vi "InterruptsGroup.vi"(0 "AnalogTriggers":T2[](array[typedef])=[{"InHysteresis"=FALSE, "OverLimit"=FALSE, "Rising"=FALSE, "Falling"=FALSE}, {"InHysteresis"=FALSE, "OverLimit"=FALSE, "Rising"=FALSE, "Falling"=FALSE}, {"InHysteresis"=FALSE, "OverLimit"=FALSE, "Rising"=FALSE, "Falling"=FALSE}, {"InHysteresis"=FALSE, "OverLimit"=FALSE, "Rising"=FALSE, "Falling"=FALSE}, {"InHysteresis"=FALSE, "OverLimit"=FALSE, "Rising"=FALSE, "Falling"=FALSE}, {"InHysteresis"=FALSE, "OverLimit"=FALSE, "Rising"=FALSE, "Falling"=FALSE}, {"InHysteresis"=FALSE, "OverLimit"=FALSE, "Rising"=FALSE, "Falling"=FALSE}, {"InHysteresis"=FALSE, "OverLimit"=FALSE, "Rising"=FALSE, "Falling"=FALSE}], 1 "DigitalInputs":bool[](array[boolean])=[FALSE, FALSE, FALSE, FALSE, FALSE, FALSE, FALSE, FALSE, FALSE, FALSE, FALSE, FALSE, FALSE, FALSE, FALSE, FALSE, FALSE, FALSE, FALSE, FALSE, FALSE, FALSE, FALSE, FALSE, FALSE, FALSE, FALSE, FALSE, FALSE, FALSE, FALSE, FALSE], 2 "SystemTime":u32, 3 "Configs":T3, 4 "Occurances":T1) -> (5 "Timestamps":T5)   [LabVIEW 2019]
uses:
  Controls/Interrupt_Timestamps.ctl
  Controls/Interrupt_Configs.ctl
  Helpers/Source.ctl
  Helpers/AnalogTriggerOutput.ctl
  Controls/Interrupt_Occurances.ctl
  <vilib>/rvi/Emulation/niFpgaSctlEmulationGetInTimedLoop.vi
  <vilib>/rvi/Emulation/niFpgaProcessEmulError.vi
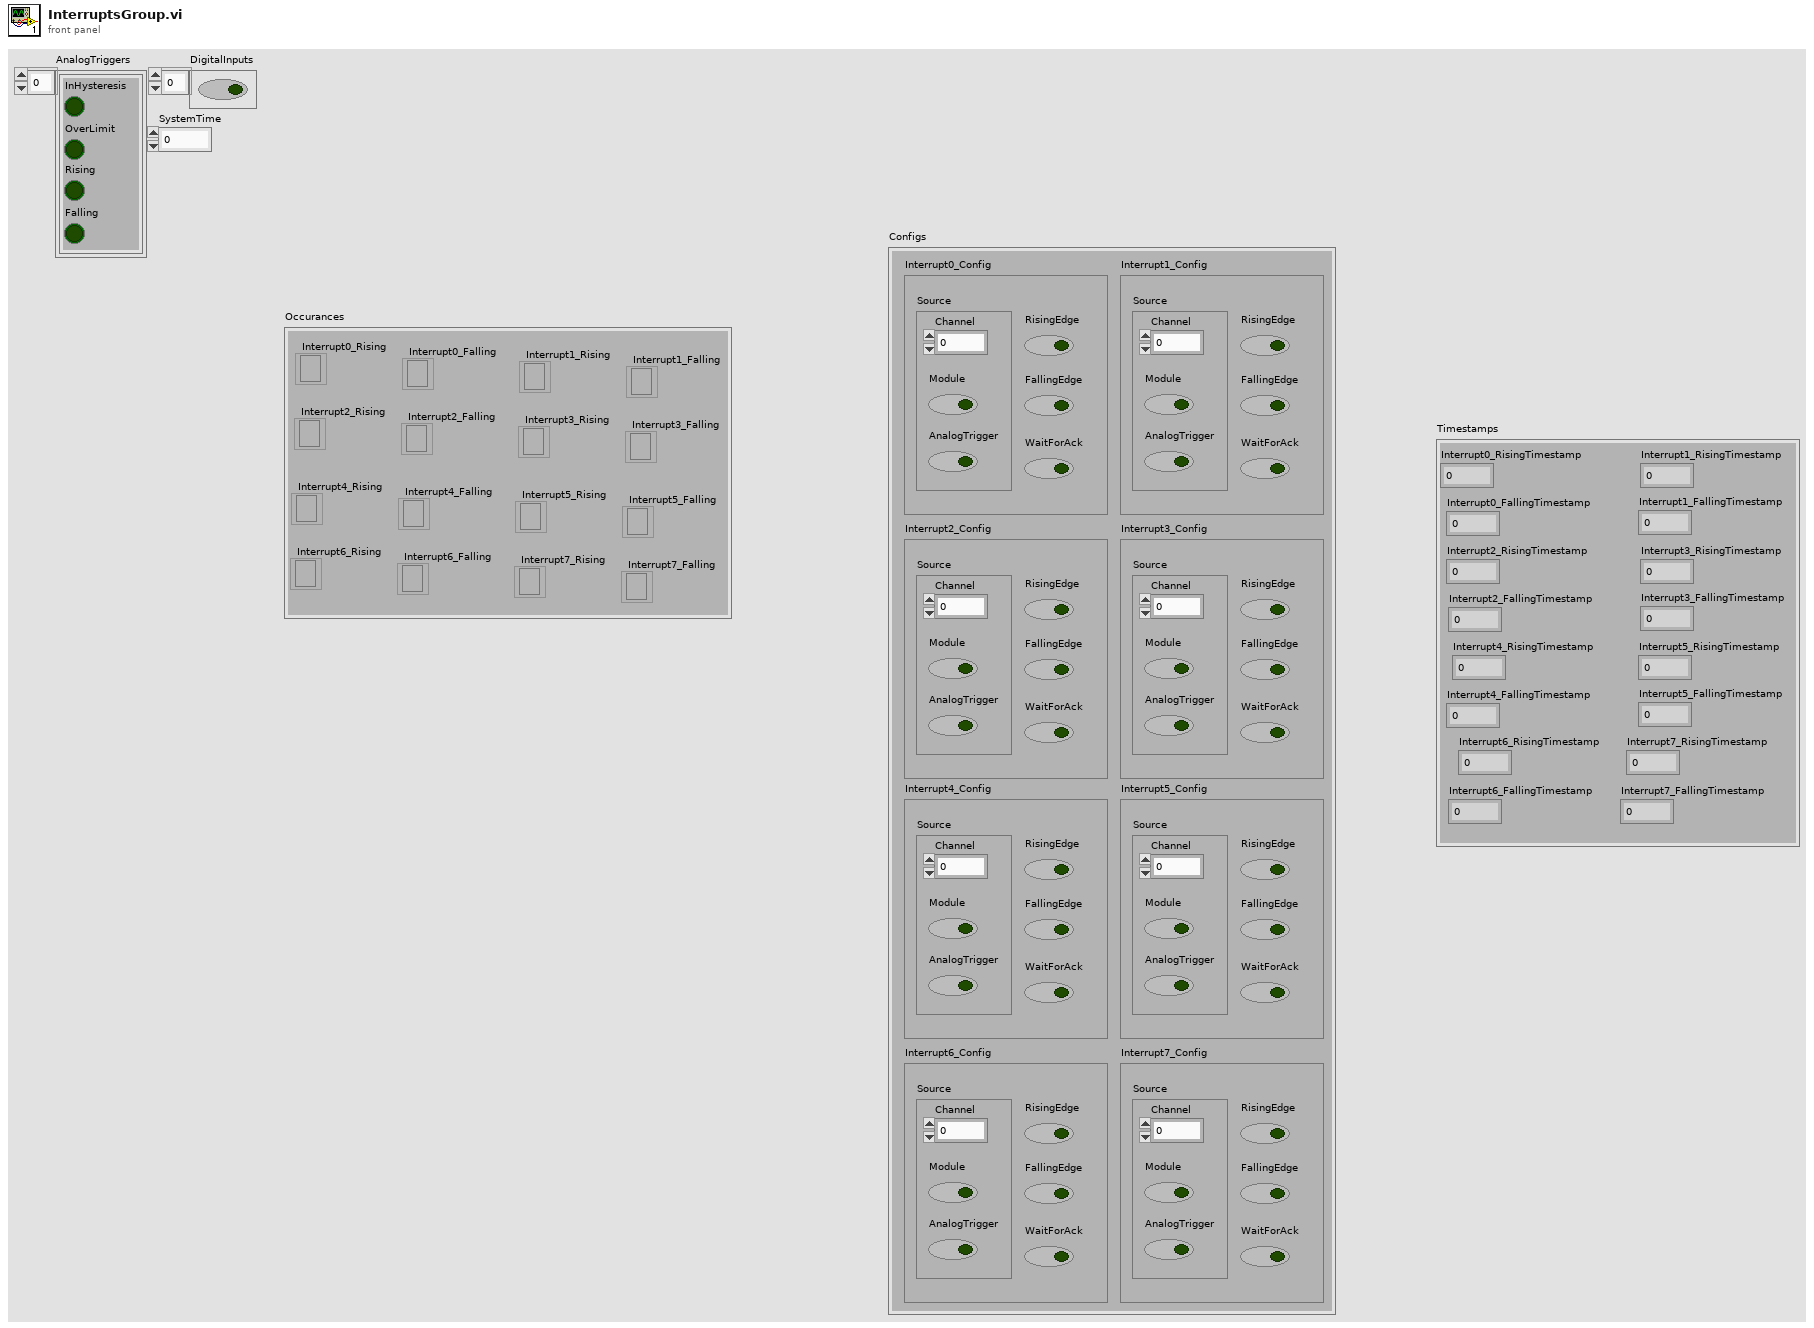
[diagram p1: front panel]
types:
  T1 = typedef "Interrupt_Occurances.ctl" = cluster{"Interrupt0_Rising":refnum<k4>, "Interrupt0_Falling":refnum<k4>, "Interrupt1_Rising":refnum<k4>, "Interrupt1_Falling":refnum<k4>, "Interrupt2_Rising":refnum<k4>, "Interrupt2_Falling":refnum<k4>, "Interrupt3_Rising":refnum<k4>, "Interrupt3_Falling":refnum<k4>, "Interrupt4_Rising":refnum<k4>, "Interrupt4_Falling":refnum<k4>, "Interrupt5_Rising":refnum<k4>, "Interrupt5_Falling":refnum<k4>, "Interrupt6_Rising":refnum<k4>, "Interrupt6_Falling":refnum<k4>, "Interrupt7_Rising":refnum<k4>, "Interrupt7_Falling":refnum<k4>}
  T2 = typedef "AnalogTriggerOutput.ctl" = cluster{"InHysteresis":bool, "OverLimit":bool, "Rising":bool, "Falling":bool}
  T3 = typedef "Interrupt_Configs.ctl" = cluster{"Interrupt0_Config":cluster{"Source":T4, "RisingEdge":bool, "FallingEdge":bool, "WaitForAck":bool}, "Interrupt1_Config":cluster{"Source":T4, "RisingEdge":bool, "FallingEdge":bool, "WaitForAck":bool}, "Interrupt2_Config":cluster{"Source":T4, "RisingEdge":bool, "FallingEdge":bool, "WaitForAck":bool}, "Interrupt3_Config":cluster{"Source":T4, "RisingEdge":bool, "FallingEdge":bool, "WaitForAck":bool}, "Interrupt4_Config":cluster{"Source":T4, "RisingEdge":bool, "FallingEdge":bool, "WaitForAck":bool}, "Interrupt5_Config":cluster{"Source":T4, "RisingEdge":bool, "FallingEdge":bool, "WaitForAck":bool}, "Interrupt6_Config":cluster{"Source":T4, "RisingEdge":bool, "FallingEdge":bool, "WaitForAck":bool}, "Interrupt7_Config":cluster{"Source":T4, "RisingEdge":bool, "FallingEdge":bool, "WaitForAck":bool}}
  T4 = typedef "Source.ctl" = cluster{"Channel":fxp<+,4,4>, "Module":bool, "AnalogTrigger":bool}
  T5 = typedef "Interrupt_Timestamps.ctl" = cluster{"Interrupt0_RisingTimestamp":u32, "Interrupt0_FallingTimestamp":u32, "Interrupt1_RisingTimestamp":u32, "Interrupt1_FallingTimestamp":u32, "Interrupt2_RisingTimestamp":u32, "Interrupt2_FallingTimestamp":u32, "Interrupt3_RisingTimestamp":u32, "Interrupt3_FallingTimestamp":u32, "Interrupt4_RisingTimestamp":u32, "Interrupt4_FallingTimestamp":u32, "Interrupt5_RisingTimestamp":u32, "Interrupt5_FallingTimestamp":u32, "Interrupt6_RisingTimestamp":u32, "Interrupt6_FallingTimestamp":u32, "Interrupt7_RisingTimestamp":u32, "Interrupt7_FallingTimestamp":u32}
  T6 = cluster{"Source":T4, "RisingEdge":bool, "FallingEdge":bool, "WaitForAck":bool}
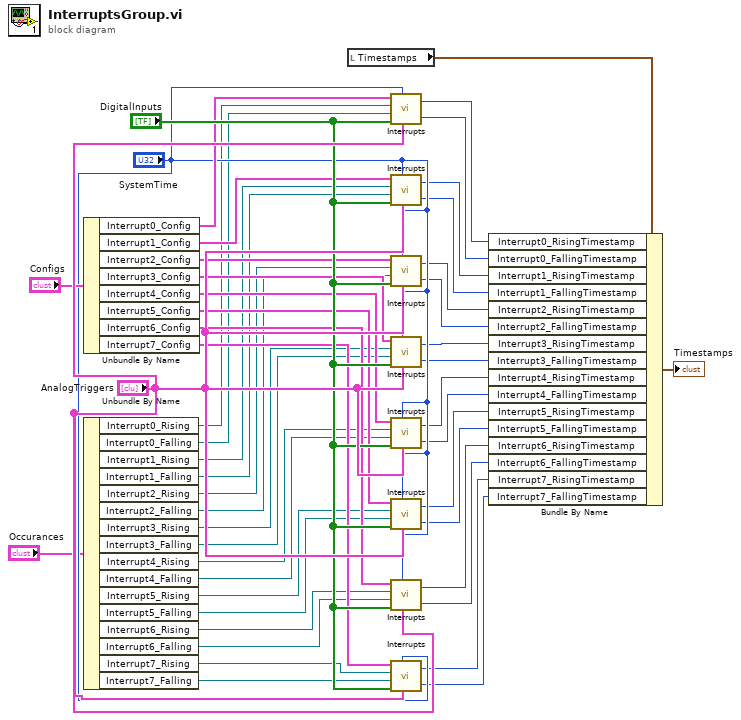
[diagram p0: block diagram]
diagram:
  n1 = Unbundle By Name("Configs") -> ("Interrupt0_Config"=w44:T6, "Interrupt1_Config"=w43:T6, "Interrupt2_Config"=w42:T6, "Interrupt3_Config"=w41:T6, "Interrupt4_Config"=w40:T6, "Interrupt5_Config"=w39:T6, "Interrupt6_Config"=w38:T6, "Interrupt7_Config"=w37:T6)
  n2 = Unbundle By Name("Occurances") -> ("Interrupt0_Rising"=w16:refnum<k4>, "Interrupt0_Falling"=w15:refnum<k4>, "Interrupt1_Rising"=w14:refnum<k4>, "Interrupt1_Falling"=w13:refnum<k4>, "Interrupt2_Rising"=w12:refnum<k4>, "Interrupt2_Falling"=w11:refnum<k4>, "Interrupt3_Rising"=w10:refnum<k4>, "Interrupt3_Falling"=w9:refnum<k4>, "Interrupt4_Rising"=w8:refnum<k4>, "Interrupt4_Falling"=w7:refnum<k4>, "Interrupt5_Rising"=w6:refnum<k4>, "Interrupt5_Falling"=w5:refnum<k4>, "Interrupt6_Rising"=w4:refnum<k4>, "Interrupt6_Falling"=w3:refnum<k4>, "Interrupt7_Rising"=w2:refnum<k4>, "Interrupt7_Falling"=w1:refnum<k4>)
  n3 = local read "Timestamps"() -> (w35:T5)
  n4 = call "Interrupts.vi"("AnalogTriggers"="AnalogTriggers", "SystemTime"="SystemTime", "DigitalInputs"="DigitalInputs", "FallingOccurance"=w15, "RisingOccurance"=w16, "Config"=w44) -> ("FallingTimestamp"=w32:u32, "RisingTimestamp"=w33:u32)
  n5 = call "Interrupts.vi"("AnalogTriggers"="AnalogTriggers", "SystemTime"="SystemTime", "DigitalInputs"="DigitalInputs", "FallingOccurance"=w13, "RisingOccurance"=w14, "Config"=w43) -> ("FallingTimestamp"=w30:u32, "RisingTimestamp"=w31:u32)
  n6 = call "Interrupts.vi"("AnalogTriggers"="AnalogTriggers", "SystemTime"="SystemTime", "DigitalInputs"="DigitalInputs", "FallingOccurance"=w11, "RisingOccurance"=w12, "Config"=w42) -> ("FallingTimestamp"=w28:u32, "RisingTimestamp"=w29:u32)
  n7 = call "Interrupts.vi"("AnalogTriggers"="AnalogTriggers", "SystemTime"="SystemTime", "DigitalInputs"="DigitalInputs", "FallingOccurance"=w9, "RisingOccurance"=w10, "Config"=w41) -> ("FallingTimestamp"=w26:u32, "RisingTimestamp"=w27:u32)
  n8 = call "Interrupts.vi"("AnalogTriggers"="AnalogTriggers", "SystemTime"="SystemTime", "DigitalInputs"="DigitalInputs", "FallingOccurance"=w7, "RisingOccurance"=w8, "Config"=w40) -> ("FallingTimestamp"=w24:u32, "RisingTimestamp"=w25:u32)
  n9 = call "Interrupts.vi"("AnalogTriggers"="AnalogTriggers", "SystemTime"="SystemTime", "DigitalInputs"="DigitalInputs", "FallingOccurance"=w5, "RisingOccurance"=w6, "Config"=w39) -> ("FallingTimestamp"=w22:u32, "RisingTimestamp"=w23:u32)
  n10 = call "Interrupts.vi"("AnalogTriggers"="AnalogTriggers", "SystemTime"="SystemTime", "DigitalInputs"="DigitalInputs", "FallingOccurance"=w3, "RisingOccurance"=w4, "Config"=w38) -> ("FallingTimestamp"=w20:u32, "RisingTimestamp"=w21:u32)
  n11 = call "Interrupts.vi"("AnalogTriggers"="AnalogTriggers", "SystemTime"="SystemTime", "DigitalInputs"="DigitalInputs", "FallingOccurance"=w1, "RisingOccurance"=w2, "Config"=w37) -> ("FallingTimestamp"=w18:u32, "RisingTimestamp"=w19:u32)
  n12 = Bundle By Name(cluster=w35, "Interrupt0_RisingTimestamp"=w33, "Interrupt0_FallingTimestamp"=w32, "Interrupt1_RisingTimestamp"=w31, "Interrupt1_FallingTimestamp"=w30, "Interrupt2_RisingTimestamp"=w29, "Interrupt2_FallingTimestamp"=w28, "Interrupt3_RisingTimestamp"=w27, "Interrupt3_FallingTimestamp"=w26, "Interrupt4_RisingTimestamp"=w25, "Interrupt4_FallingTimestamp"=w24, "Interrupt5_RisingTimestamp"=w23, "Interrupt5_FallingTimestamp"=w22, "Interrupt6_RisingTimestamp"=w21, "Interrupt6_FallingTimestamp"=w20, "Interrupt7_RisingTimestamp"=w19, "Interrupt7_FallingTimestamp"=w18) -> (→"Timestamps":T5)
